vi "test_Create FPGA Addon_Error.vi"(8 "error in (no error)":errorcluster, 11 "TestCase in":refnum<class "FPGA Addon Scripting API Unit Tests.lvclass">) -> (0 "error out":errorcluster, 3 "TestCase out":refnum<class "FPGA Addon Scripting API Unit Tests.lvclass">)   [LabVIEW 2020, in "FPGA Addon Scripting API Unit Tests.lvclass"]
uses:
  FPGA Addon Scripting API Unit Tests.lvclass
  <vilib>/addons/_JKI Toolkits/VI Tester/TestCase.llb/TestCase.lvclass
  FPGA Addon Test Class/FPGA Addon Test Class.lvclass
  APIs/Scripting API/Scripting API.lvlib
  C:/Program Files (x86)/National Instruments/LabVIEW 2020/vi.lib/addons/_JKI Toolkits/VI Tester/TestCase.llb/TestCase.lvclass
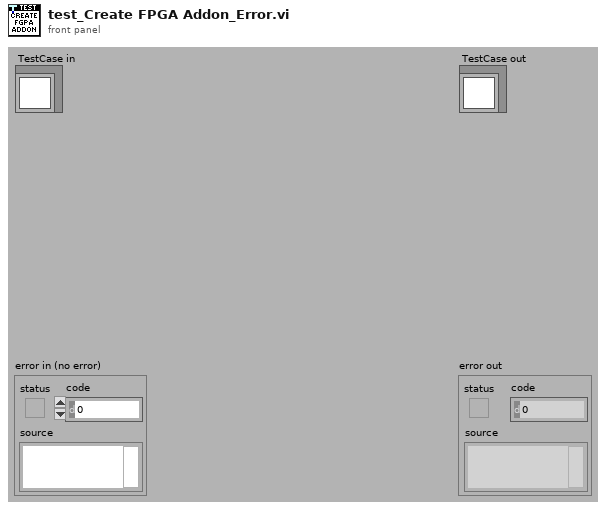
[diagram p1: front panel]
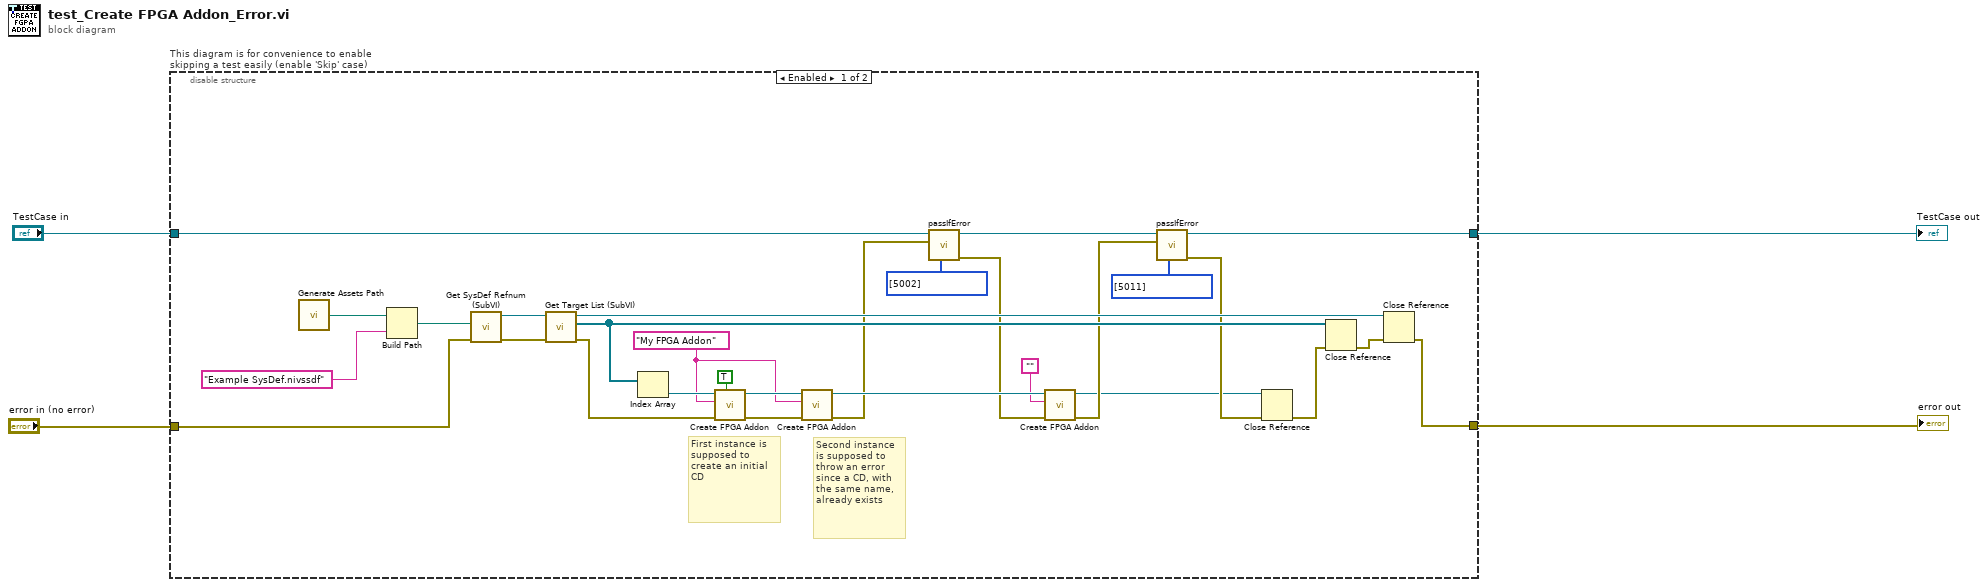
[diagram p0: block diagram]
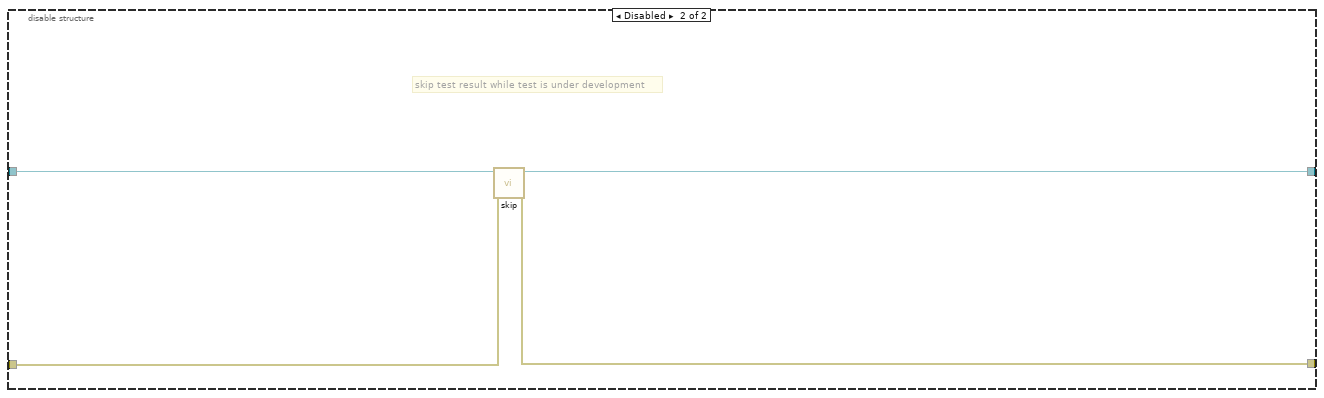
[diagram p2: hidden frame]
diagram:
  n1 = disable-structure "This diagram is for convenience to enable skipping a test easily (enable 'Skip' case)" shown="Enabled" {
    disable-tunnel: "TestCase in" -> [w17 w37]
    disable-tunnel: [w7 w35] -> w1
    disable-tunnel: [w6 w36] -> w3
    disable-tunnel: "error in (no error)" -> [w28 w34]
    frame Enabled {
      w19 = "My FPGA Addon" ("FPGA addon name")
      # "Second instance is supposed to throw an error since a CD, with the same name, already exists"
      # "First instance is supposed to create an initial CD"
      n2 = call "Generate Assets Path.vi"() -> ("Assets path"=w33:path)
      n3 = Build Path(base path=w33, name or relative path="Example SysDef.nivssdf") -> (appended path=w31:path)
      n4 = call "Get SysDef Refnum (SubVI).vi"("error in (no error)"=w28, "System Definition path"=w31) -> ("error out"=w27:errorcluster, "SysDef Refnum out"=w30:refnum<k24>)  [unwired: 8 in]
      n5 = call "Get Target List (SubVI).vi"("error in (no error)"=w27, "SysDef Refnum in"=w30) -> ("error out"=w26:errorcluster, "Target List Refnums"=w25:refnum<k24>[], "SysDef Refnum out"=w24:refnum<k24>)  [unwired: 7 in]
      n6 = Index Array(array=w25) -> (element=w29:refnum<k24>)  [unwired: 1 in]
      n7 = call "Create FPGA Addon.vi"("group scalars"=TRUE, "error in"=w26, "FPGA addon name"=w19, "target in"=w29) -> ("error out"=w21:errorcluster, "target out"=w20:refnum<k24>)  [unwired: 5 in, 1 out]
      n8 = call "Create FPGA Addon.vi"("error in"=w21, "FPGA addon name"=w19, "target in"=w20) -> ("error out"=w12:errorcluster, "target out"=w14:refnum<k24>)  [unwired: 6 in, 1 out]
      n9 = call-dynamic "passIfError.vi"("passing error codes (default = any error code)"=i32[] [5002], "error"=w12, "TestCase in"=w17) -> ("error out"=w11:errorcluster, "TestCase out"=w15:refnum<class "FPGA Addon Scripting API Unit Tests.lvclass">)  [unwired: 7 in]
      n10 = call "Create FPGA Addon.vi"("error in"=w11, "FPGA addon name"="", "target in"=w14) -> ("error out"=w10:errorcluster, "target out"=w5:refnum<k24>)  [unwired: 6 in, 1 out]
      n11 = call-dynamic "passIfError.vi"("passing error codes (default = any error code)"=i32[] [5011], "error"=w10, "TestCase in"=w15) -> ("error out"=w8:errorcluster, "TestCase out"=w7:refnum<class "FPGA Addon Scripting API Unit Tests.lvclass">)  [unwired: 7 in]
      n12 = Close Reference(reference=w5, error in (no error)=w8) -> (error out=w18:errorcluster)
      n13 = Close Reference(reference=w25, error in (no error)=w18) -> (error out=w23:errorcluster)
      n14 = Close Reference(reference=w24, error in (no error)=w23) -> (error out=w6:errorcluster)
    }
    frame Disabled {
      # "skip test result while test is under development"
      n15 = call <vilib>:"skip.vi"("error in (no error)"=w34, "TestCase in"=w37) -> ("error out"=w36:errorcluster, "TestCase out"=w35:refnum<class "FPGA Addon Scripting API Unit Tests.lvclass">)  [unwired: 8 in]
    }
  }
  "error out" <- w3
  "TestCase out" <- w1
